vi "IniQueue.vi"() -> (0 "error out":errorcluster, 3 "Cluster":T1)   [LabVIEW 2017]
uses:
  Event clusterr.ctl
  EventMsg.ctl
  Sequence cluster.ctl
  SequenceMsg.ctl
  LowLevel cluster.ctl
  LowLevelMsg.ctl
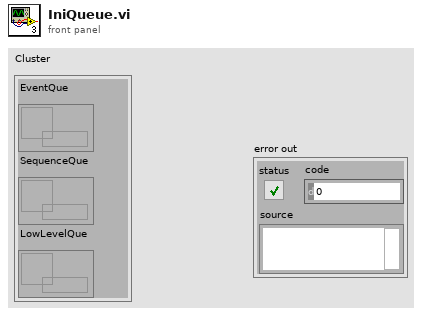
[diagram p1: front panel]
types:
  T1 = cluster{"EventQue":refnum<queue>, "SequenceQue":refnum<queue>, "LowLevelQue":refnum<queue>}
  T2 = typedef "LowLevel cluster.ctl" = cluster{"LowLevelMsg":T3, "LowLevel string":string}
  T3 = typedef "LowLevelMsg.ctl" = enum16{"ResetArduinoState", "Init", "Halt", "SetArduinoState", "RunStopSigGen", "Error"}
  T4 = typedef "Event clusterr.ctl" = cluster{"EventMsg":T5, "Event string":string}
  T5 = typedef "EventMsg.ctl" = enum16{"Init", "Halt", "Listen"}
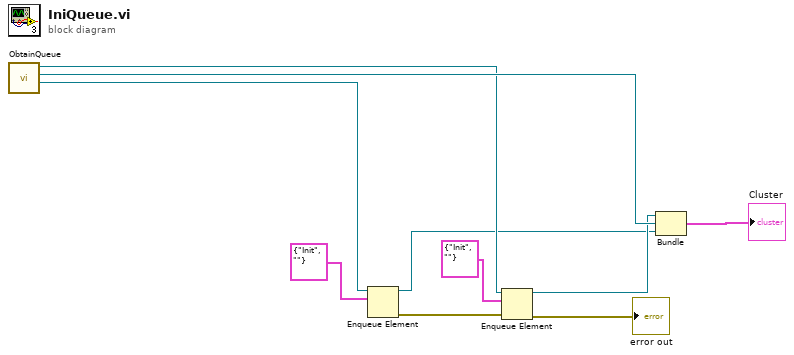
[diagram p0: block diagram]
diagram:
  n1 = call "ObtainQueue.vi"() -> ("LowLevelQue"=w3:refnum<queue>, "SequenceQue"=w9:refnum<queue>, "EventQue"=w6:refnum<queue>)  [unwired: 8 in, 1 out]
  n2 = Enqueue Element(queue=w3, element=T2 {"LowLevelMsg"=enum."Init", "LowLevel string"=""}) -> (queue out=w1:refnum<queue>, error out=w4:errorcluster)  [unwired: 2 in, 1 out]
  n3 = Enqueue Element(queue=w6, element=T4 {"EventMsg"=enum."Init", "Event string"=""}, error in (no error)=w4) -> (queue out=w8:refnum<queue>, error out=→"error out":errorcluster)  [unwired: 1 in, 1 out]
  n4 = Bundle("EventQue"=w8, "SequenceQue"=w9, "LowLevelQue"=w1) -> (→"Cluster":T1)  [unwired: 1 in]
